vi "Aero_Chilled_Water_PID.vi"(1 "Tweak in working section demanded temp":dbl, 2 "Present Value":dbl=15.0 format="%.2f", 3 "Reset PID":bool, 4 "Setpoint":dbl=15.0 format="%.2f") -> (0 "Dem Output":dbl format="%.2f")   [LabVIEW 2017]
uses:
  <vilib>/Analysis/NI_AALPro.lvlib
panel:
  out "Derivative":dbl(graph)
  out "Integral":dbl(graph)
  out "Proportional":dbl(graph)
  out "Error":dbl(graph)
  in  "O/P deadband":dbl=1.0 format="%.2f"
  in  "Kp Deadband":dbl format="%.2f"
  in  "Derivative History":i32=4
  out "deadbanded error":dbl format="%.2f"
  in  "P":bool=TRUE
  in  "D":bool=TRUE
  in  "I":bool=TRUE
  in  "Manual Demand":dbl min=0.0 max=100.0 format="%.2f"
  in  "Manual Override":bool
  out "Control Sum":dbl format="%.2f"
  out "error differential":dbl format="%.5f"
  in  "Kd":dbl=500.0 format="%.2f"
  in  "Ki":dbl=0.571 format="%.2f"
  in  "Kp":dbl=15.0 format="%.2f"
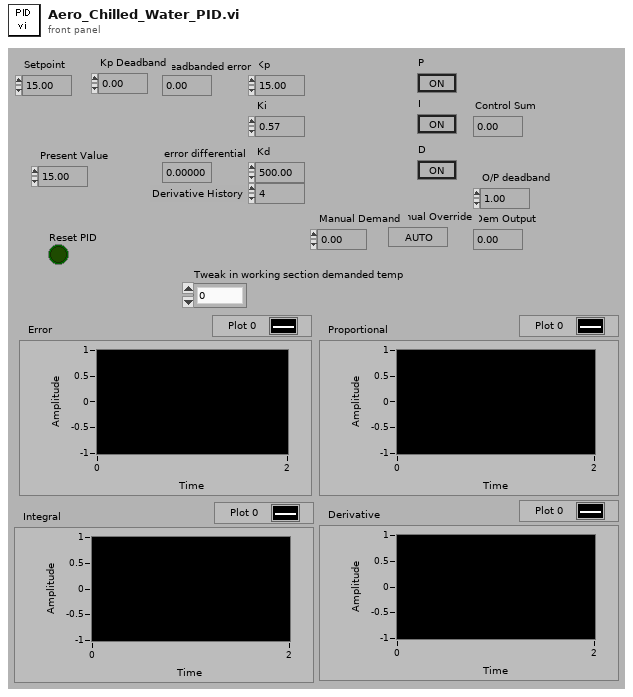
[diagram p1: front panel]
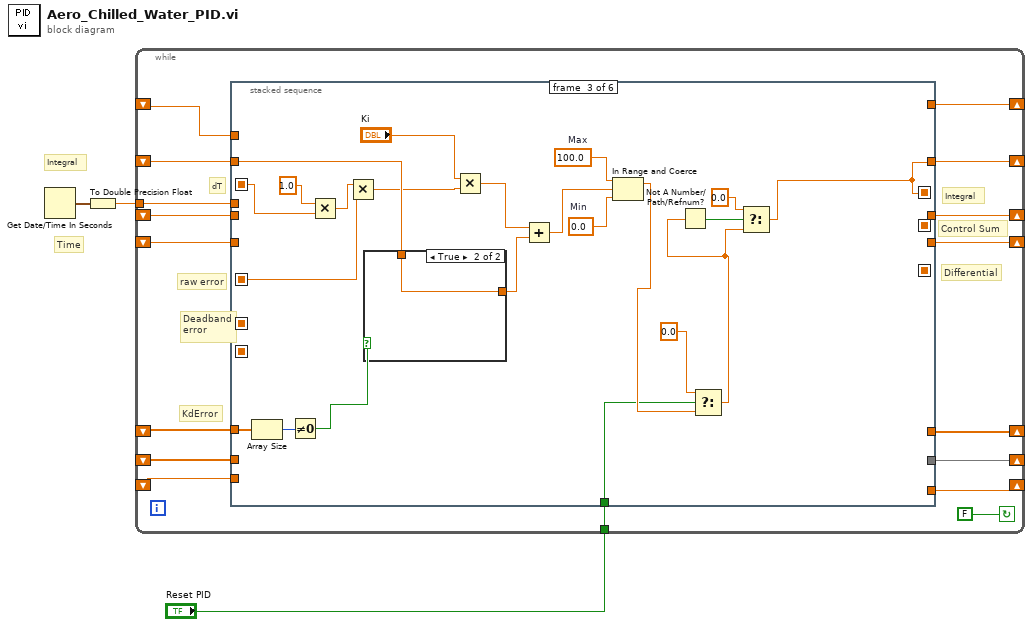
[diagram p0: block diagram]
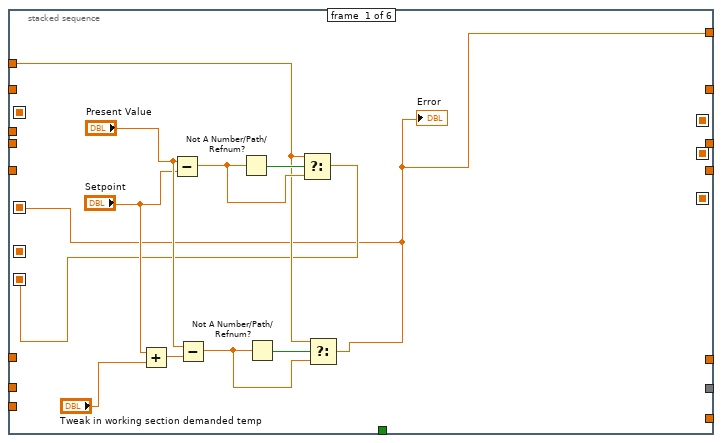
[diagram p2: hidden frame]
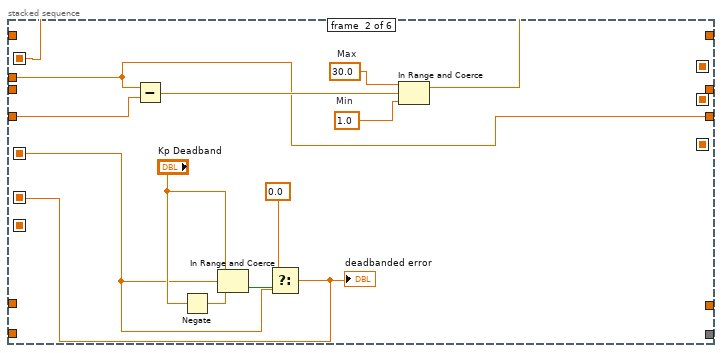
[diagram p3: hidden frame]
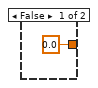
[diagram p4: hidden frame]
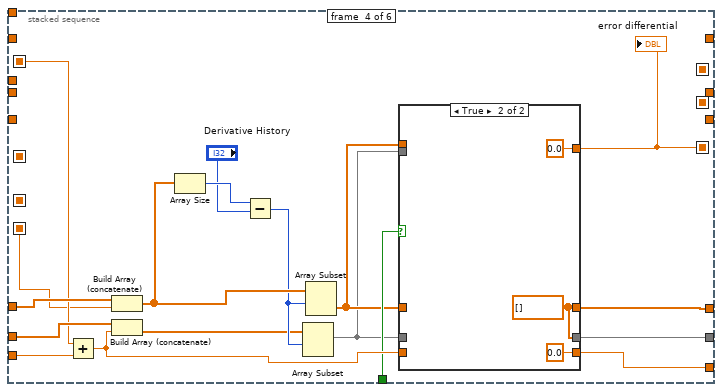
[diagram p5: hidden frame]
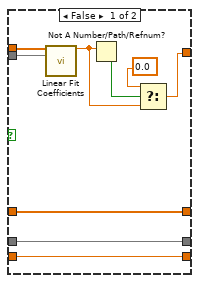
[diagram p6: hidden frame]
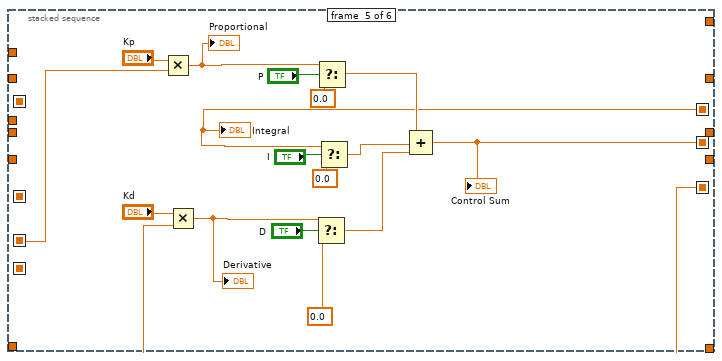
[diagram p7: hidden frame]
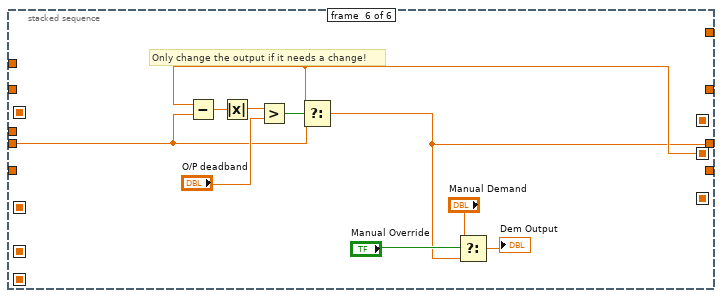
[diagram p8: hidden frame]
diagram:
  # "Integral"
  # "Time"
  n1 = Get Date/Time In Seconds() -> (seconds since 1Jan1904=w2:timestamp)
  n2 = To Double Precision Float(number=w2) -> (double precision float=w3:dbl)
  n3 = while {
    shift-left: _ -> [w7]
    shift-right: [w6] -> _
    shift-left: _ -> [w9]
    shift-right: [w8] -> _
    shift-left: _ -> [w11]
    shift-right: [w10] -> _
    tunnel: w3 -> [w16]
    shift-left: _ -> [w13]
    shift-right: [w12] -> _
    shift-left: _ -> [w15]
    shift-right: [w14] -> _
    shift-left: _ -> [w17]
    shift-right: [w18] -> _
    shift-left: _ -> [w20]
    shift-right: [w19] -> _
    tunnel: "Reset PID" -> [w4]
    stop <- FALSE continue-if-true
    # "KdError"
    # "Control Sum"
    # "raw error"
    # "Differential"
    # "Integral"
    # "Deadband\nerror"
    # "dT"
    n4 = stacked-sequence {
      seq-local: [_ w32 _ _ _ _] -> [_ _ w55 w77 _ _]
      seq-local: [_ w41 _ _ _ _] -> [_ _ _ _ w102 _]
      seq-local: [_ _ _ w78 _ _] -> [_ _ _ _ w101 _]
      seq-local: [_ _ w48 _ _ _] -> [_ _ _ _ w98 _]
      seq-local: [w21 _ _ _ _ _] -> [_ w33 w63 _ _ _]
      seq-local: [_ _ _ _ w105 _] -> [_ _ _ _ _ w118]
      seq-local: [w22 _ _ _ _ _] -> [_ _ _ w75 _ _]
      tunnel: w20 -> [_ w38 _ _ _ _]
      tunnel: [_ w36 _ _ _ _] -> w19
      tunnel: [_ _ w48 _ _ _] -> w18
      tunnel: w17 -> [_ _ w53 _ _ _]
      tunnel: w16 -> [_ w36 _ _ _ _]
      tunnel: w15 -> [_ _ w62 w85 _ _]
      tunnel: [_ _ _ w71 _ _] -> w14
      tunnel: w13 -> [_ _ _ w84 _ _]
      tunnel: [_ _ _ w69 _ _] -> w12
      tunnel: w11 -> [_ _ _ _ _ w116]
      tunnel: [_ _ _ _ _ w115] -> w10
      tunnel: w9 -> [_ _ _ w76 _ _]
      tunnel: [_ _ _ w74 _ _] -> w8
      tunnel: w7 -> [w27 _ _ _ _ _]
      tunnel: [w21 _ _ _ _ _] -> w6
      tunnel: w4 -> [_ _ w49 w72 _ _]
      frame #0 {
        n5 = Add(x="Setpoint", y="Tweak in working section demanded temp") -> (x+y=w23:dbl)
        n6 = Subtract(x="Present Value", y="Setpoint") -> (x-y=w30:dbl)
        n7 = Subtract(x="Present Value", y=w23) -> (x-y=w29:dbl)
        n8 = Not A Number/Path/Refnum?(number/path/refnum=w30) -> (NaN/Path/Refnum?=w31:bool)
        n9 = Not A Number/Path/Refnum?(number/path/refnum=w29) -> (NaN/Path/Refnum?=w28:bool)
        n10 = Select(t=w27, s=w31, f=w30) -> (s? t:f=w22:dbl)
        n11 = Select(t=w27, s=w28, f=w29) -> (s? t:f=w21:dbl)
        "Error" <- w21
      }
      frame #1 {
        w39 = 1.0  # Min
        w40 = 30.0  # Max
        n12 = Subtract(x=w36, y=w38) -> (x-y=w37:dbl)
        n13 = Negate(x="Kp Deadband") -> (-x=w35:dbl)
        n14 = In Range and Coerce(upper limit="Kp Deadband", x=w33, lower limit=w35) -> (In Range?=w42:bool)  [unwired: 1 out]
        n15 = Select(t=0.0, s=w42, f=w33) -> (s? t:f=w41:dbl)
        "deadbanded error" <- w41
        n16 = In Range and Coerce(upper limit=w40, x=w37, lower limit=w39) -> (coerced(x)=w32:dbl)  [unwired: 1 out]
      }
      frame #2 {
        w65 = 0.0  # Min
        w47 = 100.0  # Max
        n17 = Array Size(array=w62) -> (size(s)=w61:i32)
        n18 = Not Equal To 0?(x=w61) -> (x != 0?=w60:bool)
        n19 = Multiply(x=1.0, y=w55) -> (x*y=w54:dbl)
        n20 = Multiply(x=w54, y=w63) -> (x*y=w46:dbl)
        n21 = case shown="True" w60 {
          tunnel: [0.0 ("Min") w67] -> w59
          tunnel: w53 -> [_ w67]
          frame False {
          }
          frame True {
          }
        }
        n22 = Multiply(x="Ki", y=w46) -> (x*y=w44:dbl)
        n23 = Add(x=w44, y=w59) -> (x+y=w64:dbl)
        n24 = In Range and Coerce(upper limit=w47, x=w64, lower limit=w65) -> (coerced(x)=w51:dbl)  [unwired: 1 out]
        n25 = Select(t=0.0, s=w49, f=w51) -> (s? t:f=w50:dbl)
        n26 = Not A Number/Path/Refnum?(number/path/refnum=w50) -> (NaN/Path/Refnum?=w57:bool)
        n27 = Select(t=0.0, s=w57, f=w50) -> (s? t:f=w48:dbl)
      }
      frame #3 {
        n28 = Add(x=w77, y=w76) -> (x+y=w73:dbl)
        n29 = Build Array (concatenate)(w85, w75) -> (w81:dbl[])
        n30 = Build Array (concatenate)(w84, w73) -> (w79:dbl[])
        n31 = Array Size(array=w81) -> (size(s)=w83:i32)
        n32 = Subtract(x=w83, y="Derivative History") -> (x-y=w80:i32)
        n33 = Array Subset(array=w79, index=w80) -> (w68:dbl[])  [unwired: 1 in]
        n34 = Array Subset(array=w81, index=w80) -> (w70:dbl[])  [unwired: 1 in]
        n35 = case shown="True" w72 {
          tunnel: w70 -> [w94 _]
          tunnel: [w88 0.0 ("slope")] -> w78
          tunnel: w68 -> [w93 _]
          tunnel: [w89 0.0] -> w74
          tunnel: w73 -> [w89 _]
          tunnel: [w87 w96] -> w71
          tunnel: w70 -> [w87 _]
          tunnel: [w86 w96] -> w69
          tunnel: w68 -> [w86 _]
          frame False {
            n36 = call <vilib>:"Linear Fit Coefficients.vi"("Y"=w94, "X"=w93) -> ("slope"=w90:dbl)  [unwired: 3 in, 10 out]
            n37 = Not A Number/Path/Refnum?(number/path/refnum=w90) -> (NaN/Path/Refnum?=w92:bool)
            n38 = Select(t=0.0 ("f"), s=w92, f=w90) -> (s? t:f=w88:dbl)
          }
          frame True {
            w96 = dbl[] []
          }
        }
        "error differential" <- w78
      }
      frame #4 {
        n39 = Multiply(x="Kp", y=w102) -> (x*y=w99:dbl)
        "Proportional" <- w99
        n40 = Multiply(x="Kd", y=w101) -> (x*y=w100:dbl)
        "Derivative" <- w100
        n41 = Select(t=w100, s="D", f=0.0) -> (s? t:f=w107:dbl)
        n42 = Select(t=w99, s="P", f=0.0) -> (s? t:f=w113:dbl)
        n43 = Select(t=w98, s="I", f=0.0) -> (s? t:f=w106:dbl)
        n44 = Compound Arithmetic op=ADD(w113, w106, w107) -> (w105:dbl)
        "Control Sum" <- w105
        "Integral" <- w98
      }
      frame #5 {
        # "Only change the output if it needs a change!"
        n45 = Subtract(x=w118, y=w116) -> (x-y=w121:dbl)
        n46 = Absolute Value(x=w121) -> (abs(x)=w120:dbl)
        n47 = Greater?(x=w120, y="O/P deadband") -> (0:w119:bool)
        n48 = Select(t=w118, s=w119, f=w116) -> (s? t:f=w115:dbl)
        n49 = Select(t="Manual Demand", s="Manual Override", f=w115) -> (s? t:f=→"Dem Output":dbl)
      }
    }
  }
